vi "checksum.vi"(8 "error in (no error)":errorcluster, 10 "input":string, 11 "DeviceInterface in":refnum<class "DeviceInterface.lvclass">) -> (0 "error out":errorcluster, 2 "output":string, 3 "DeviceInterface out":refnum<class "DeviceInterface.lvclass">)   [LabVIEW 2013, in "DeviceInterface.lvclass"]
uses:
  DeviceInterface.lvclass
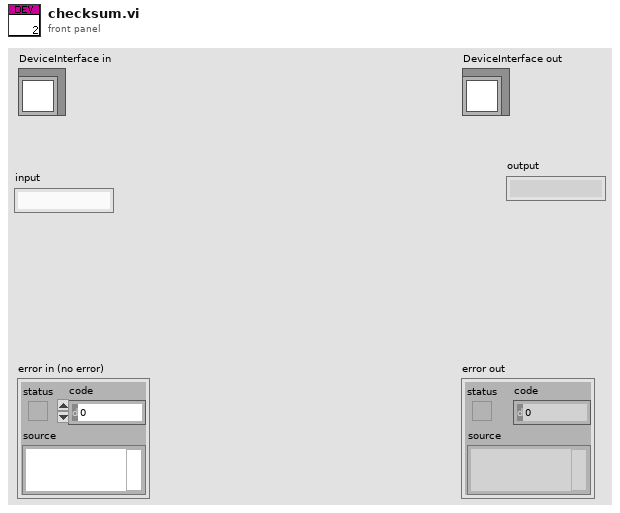
[diagram p1: front panel]
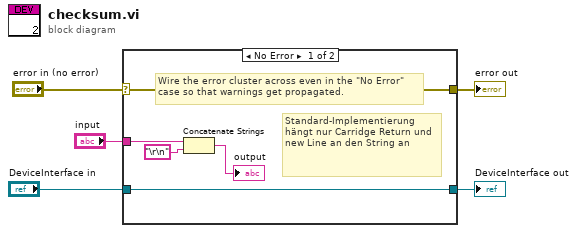
[diagram p0: block diagram]
diagram:
  n1 = case shown="No Error" "error in (no error)" {
    selector: "error in (no error)" -> [w9 w12]
    tunnel: [w9 w12] -> w4
    tunnel: [w10 w11] -> w2
    tunnel: "DeviceInterface in" -> [w10 w11]
    tunnel: "input" -> [w8 _]
    frame No Error {
      # "Standard-Implementierung hängt nur Carridge Return und new Line an den String an"
      # "Wire the error cluster across even in the \"No Error\"\ncase so that warnings get propagated."
      n2 = Concatenate Strings(w8, "\r\n") -> (→"output":string)
    }
    frame Error {
    }
  }
  "error out" <- w4
  "DeviceInterface out" <- w2
